vi "kvCanSetBusOutputControl.vi"(2 "error in (no error)":errorcluster, 3 "Silent":bool caption="Normal", 4 "Channel Handle (input only)":i32) -> (0 "error out":errorcluster, 1 "Channel Handle (ouput only)":i32)   [LabVIEW 2022 SP3]
doc: "This function sets the driver type for a CAN controller. This corresponds loosely to the bus output control register in the CAN controller, hence the name of this function. CANLIB32 does not allow for direct manipulation of the bus output control register; instead, symbolic constants are used to select the desired driver type. \n\nDon't confuse the CAN controller driver type with the bus driver type. The CAN controller is not connected directly to the CAN bus; instead, it is connected to a bus transceiver circuit which interfaces directly to the bus. The \"CAN controller driver type\" we are talking about here refers to the mode which the CAN controller uses to drive the bus transceiver circuit. CANLIB supports two different modes:\n\nNormal mode, which is.. well.. the normal mode. \n\nSilent mode, where the CAN controller does not send anything on the bus, not even ACK bits. Reception, however, works as usual. \nNote that Silent Mode is not supported by all CAN controllers."
uses:
  canlib32.dll
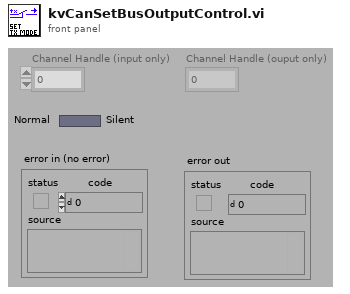
[diagram p1: front panel]
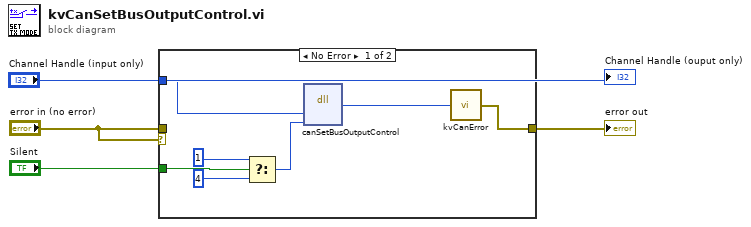
[diagram p0: block diagram]
diagram:
  n1 = case shown="No Error" "error in (no error)" {
    tunnel: "Channel Handle (input only)" -> [w11 _]
    tunnel: "error in (no error)" -> [_ w12]
    tunnel: [w9 w12] -> w3
    tunnel: "Silent" -> [w7 _]
    frame No Error {
      n2 = Select(t=1, s=w7, f=4) -> (s? t:f=w8:i32)
      n3 = dll-call lib="canlib32.dll" fn="canSetBusOutputControl" label="Call canSetBusOutputControl"("channelHandle"=w11, "drivertype"=w8) -> (w10:u32)  [unwired: 5 in, 2 out]
      n4 = call "kvCanError.vi"("error code"=w10) -> ("error out"=w9:errorcluster)
    }
    frame Error {
    }
  }
  "error out" <- w3
  "Channel Handle (ouput only)" <- "Channel Handle (input only)"
